vi "F to C (1D dbl).vi"(1 "F":dbl[](array[numeric])) -> (0 "C":dbl[](array[numeric]))   [LabVIEW 2012, in "Temp Converter.lvlib"]
doc: "<B>输入端子C</B>: 输入华氏温度。\n<B>输出端子C</B>: 输出摄氏温度。\n\n公式：C=(F-32)*5/9.\n创建者：CSXCS_366"
uses:
  Temp Converter.lvlib
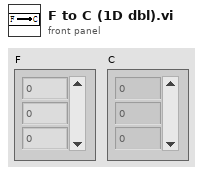
[diagram p1: front panel]
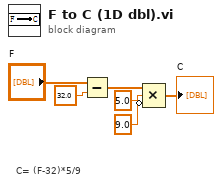
[diagram p0: block diagram]
diagram:
  # "C= (F-32)*5/9"
  n1 = Subtract(x="F", y=32.0 ("x")) -> (x-y=w3:dbl[])
  n2 = Compound Arithmetic op=MULTIPLY(w3, 5.0 ("y"), invert 9.0 ("值")) -> (→"C":dbl[])
